vi "Gate Delay Manager.vi"(0 "Gate Delay Actions":T2, 2 "Gate Delay Names":T1, 11 "Delay Time In (ns)":dbl format="%#_13g") -> (4 "Laser Delay (ns)":dbl, 8 "Window Delay (ns)":dbl, 15 "Window Width (ns)":dbl)   [LabVIEW 2016]
uses:
  Gate Delay Type Defs/Gate Delay Actions.ctl
  Gate Delay Type Defs/Board Names.ctl
  Gate Delay Type Defs/Gate Delay Notifier Element.ctl
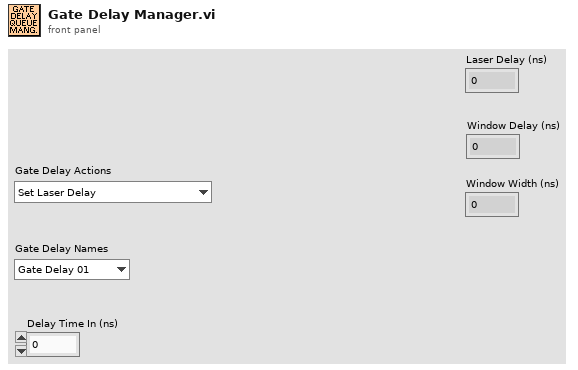
[diagram p1: front panel]
types:
  T1 = typedef "Board Names.ctl" = enum16{"Gate Delay 01", "Gate Delay 02"}
  T2 = typedef "Gate Delay Actions.ctl" = enum16{"Set Laser Delay", "Set Window Delay", "Set Window Width", "Get Delays", "Set Default Delays", "Restore Defaults", "Quit"}
  T3 = typedef "Gate Delay Notifier Element.ctl" = cluster{"Gate Delay Actions":T2, "Laser Delay":dbl, "Window Delay":dbl, "Window Width":dbl, "Command Received?":bool}
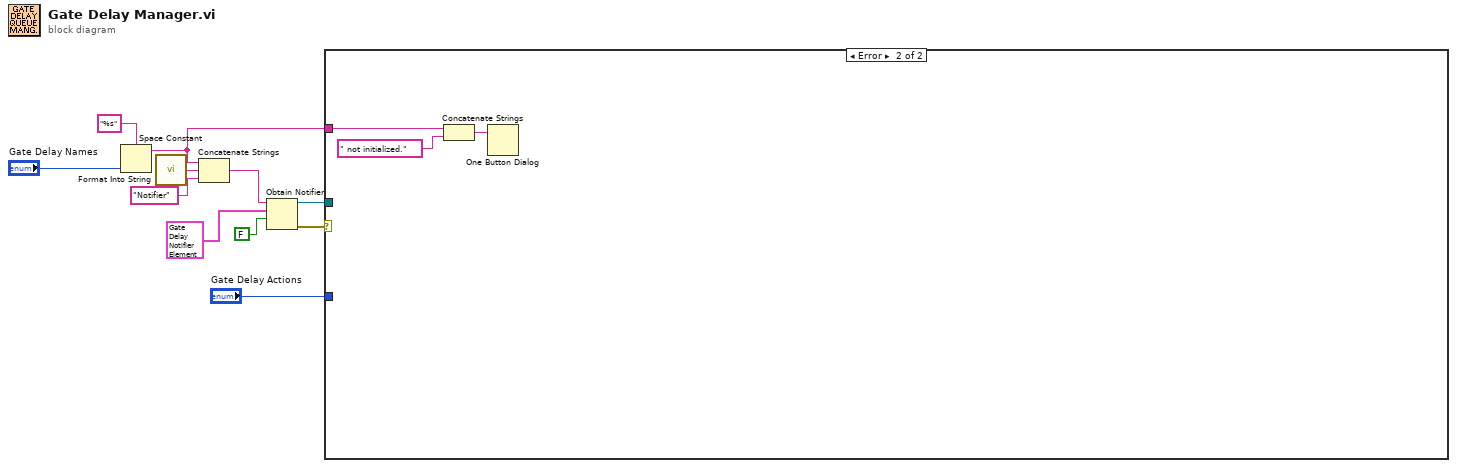
[diagram p0: block diagram]
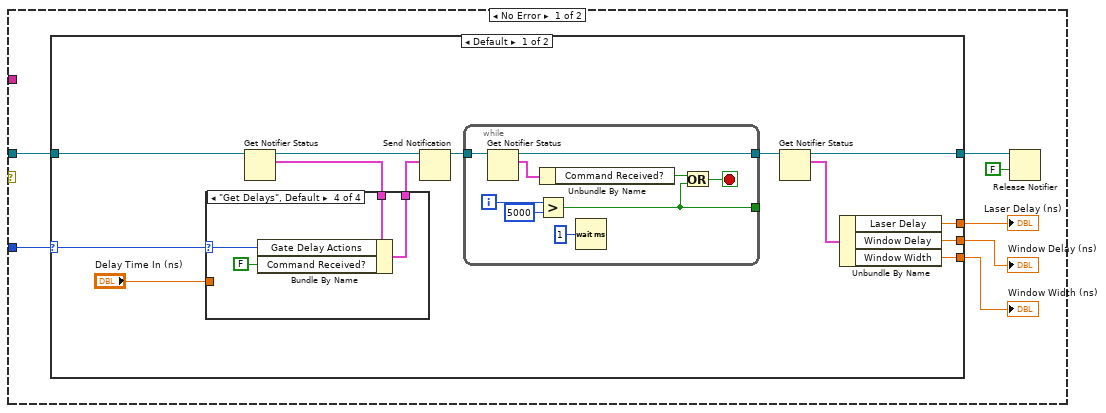
[diagram p2: hidden frame]
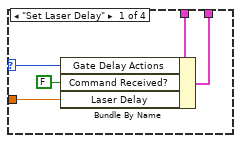
[diagram p3: hidden frame]
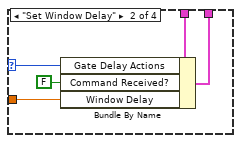
[diagram p4: hidden frame]
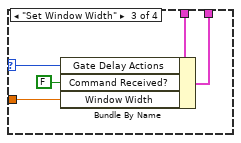
[diagram p5: hidden frame]
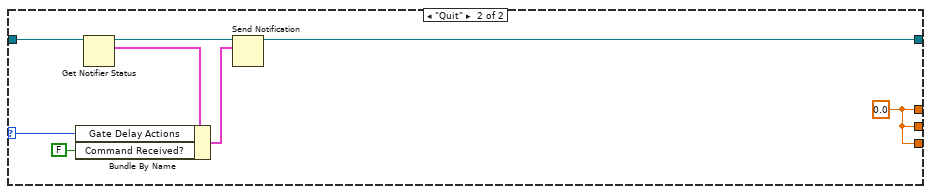
[diagram p6: hidden frame]
diagram:
  n1 = Format Into String(format string="%s", "Gate Delay Names") -> (resulting string=w2:string)  [unwired: 2 in, 1 out]
  n2 = call <vilib>:"Space Constant.vi"() -> ("String"=w10:string)
  n3 = Concatenate Strings(w2, w10, "Notifier" ("string")) -> (w7:string)
  n4 = Obtain Notifier(name (unnamed)=w7, notification data type=T3 {"Gate Delay Actions"=enum."Set Laser Delay", "Laser Delay"=0.0, "Window Delay"=0.0, "Window Width"=0.0, "Command Received?"=FALSE} ("Gate Delay Notifier Element"), create if not found? (T)=FALSE) -> (notifier out=w3:refnum<notifier>, error out=w5:errorcluster)  [unwired: 1 in, 1 out]
  n5 = case shown="Error" w5 {
    tunnel: w3 -> [w18 _]
    tunnel: w2 -> [_ w68]
    tunnel: "Gate Delay Actions" -> [w17 _]
    frame No Error {
      n6 = case shown="Default" w17 {
        selector: w17 -> [w23 w65]
        tunnel: w18 -> [w31 w66]
        tunnel: [w22 w61] -> w15
        tunnel: [w21 w60] -> w14
        tunnel: [w20 w60] -> w13
        tunnel: [w19 w60] -> w12
        frame Default {
          n7 = Get Notifier Status(notifier=w31) -> (notifier out=w29:refnum<notifier>, current notification=w30:T3)  [unwired: 1 in, 3 out]
          n8 = case shown="\"Get Delays\", Default" w23 {
            selector: w23 -> [w33 w38 w43 w47]
            tunnel: w30 -> [w36 w41 w46 w50]
            tunnel: [w34 w39 w44 w48] -> w28
            tunnel: "Delay Time In (ns)" -> [w32 w37 w42 _]
            frame "Set Laser Delay" {
              n9 = Bundle By Name(cluster=w36, "Gate Delay Actions"=w33, "Command Received?"=FALSE, "Laser Delay"=w32) -> (w34:T3)
            }
            frame "Set Window Delay" {
              n10 = Bundle By Name(cluster=w41, "Gate Delay Actions"=w38, "Command Received?"=FALSE, "Window Delay"=w37) -> (w39:T3)
            }
            frame "Set Window Width" {
              n11 = Bundle By Name(cluster=w46, "Gate Delay Actions"=w43, "Command Received?"=FALSE, "Window Width"=w42) -> (w44:T3)
            }
            frame "Get Delays", Default {
              n12 = Bundle By Name(cluster=w50, "Gate Delay Actions"=w47, "Command Received?"=FALSE) -> (w48:T3)
            }
          }
          n13 = Send Notification(notification=w28, notifier=w29) -> (notifier out=w27:refnum<notifier>)  [unwired: 1 in, 1 out]
          n14 = while {
            tunnel: w27 -> [w59]
            tunnel: [w57] -> w26
            tunnel: [w51] -> _
            i -> [w56]
            stop <- w53 stop-if-true
            n15 = Get Notifier Status(notifier=w59) -> (notifier out=w57:refnum<notifier>, current notification=w58:T3)  [unwired: 1 in, 3 out]
            n16 = Greater?(x=w56, y=5000) -> (0:w51:bool)
            n17 = Unbundle By Name(w58) -> ("Command Received?"=w54:bool)
            n18 = Wait (ms)(milliseconds to wait=u32 1) -> ()  [unwired: 1 out]
            n19 = Or(x=w54, y=w51) -> (x .or. y?=w53:bool)
          }
          n20 = Get Notifier Status(notifier=w26) -> (notifier out=w22:refnum<notifier>, current notification=w24:T3)  [unwired: 1 in, 3 out]
          n21 = Unbundle By Name(w24) -> ("Laser Delay"=w21:dbl, "Window Delay"=w20:dbl, "Window Width"=w19:dbl)
        }
        frame "Quit" {
          w60 = 0.0 ("Laser Delay")
          n22 = Get Notifier Status(notifier=w66) -> (notifier out=w67:refnum<notifier>, current notification=w64:T3)  [unwired: 1 in, 3 out]
          n23 = Bundle By Name(cluster=w64, "Gate Delay Actions"=w65, "Command Received?"=FALSE) -> (w63:T3)
          n24 = Send Notification(notification=w63, notifier=w67) -> (notifier out=w61:refnum<notifier>)  [unwired: 1 in, 1 out]
        }
      }
      "Laser Delay (ns)" <- w14
      "Window Delay (ns)" <- w13
      "Window Width (ns)" <- w12
      n25 = Release Notifier(notifier=w15, force destroy? (F)=FALSE) -> ()  [unwired: 1 in, 3 out]
    }
    frame Error {
      n26 = Concatenate Strings(w68, " not initialized." ("message")) -> (w70:string)
      n27 = One Button Dialog(message=w70) -> ()  [unwired: 1 in, 1 out]
    }
  }
